vi "bt.vi"(2 "system_stage":string, 8 "LabVIEW Web Service Request":refnum<class "Web Request.lvclass">) -> (1 "position":string, 4 "reduce_head_movement":bool, 7 "congrats_level":string, 9 "therapy_stage":string, 10 "home":string, 13 "target":string, 14 "EEG_Impedances":string, 17 "EOG_Impedances":string, 18 "VI_running":string, 19 "trial_number":string, 26 "VI_stream":string)   [LabVIEW 2020]
uses:
  <vilib>/wsapi/Web Request.lvclass
  Global 1.vi
panel:
  # "Use the Web Service Request input terminal to call the VIs on the Web Services palette. Do not remove it from the connector pane unless you don't need access to the palette."
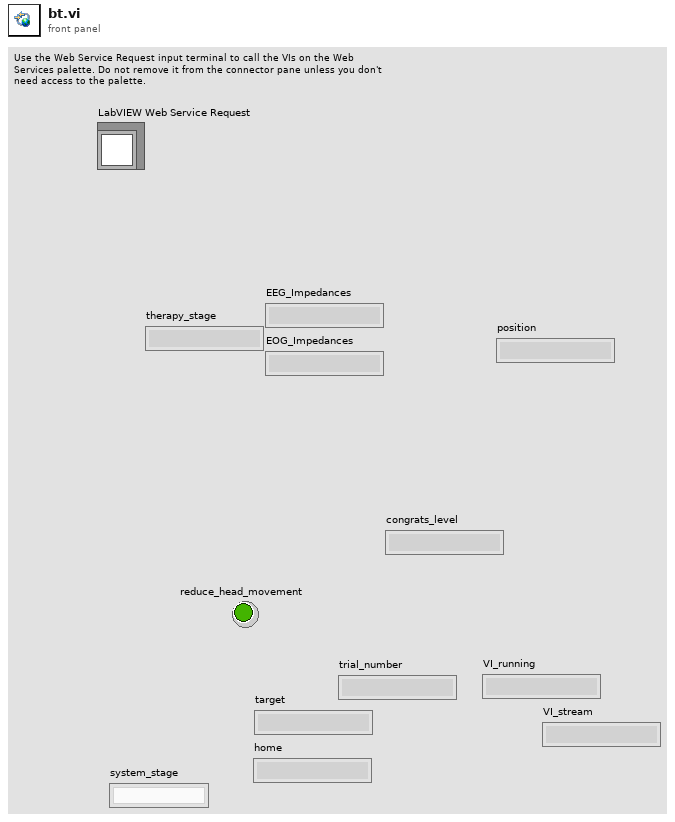
[diagram p1: front panel]
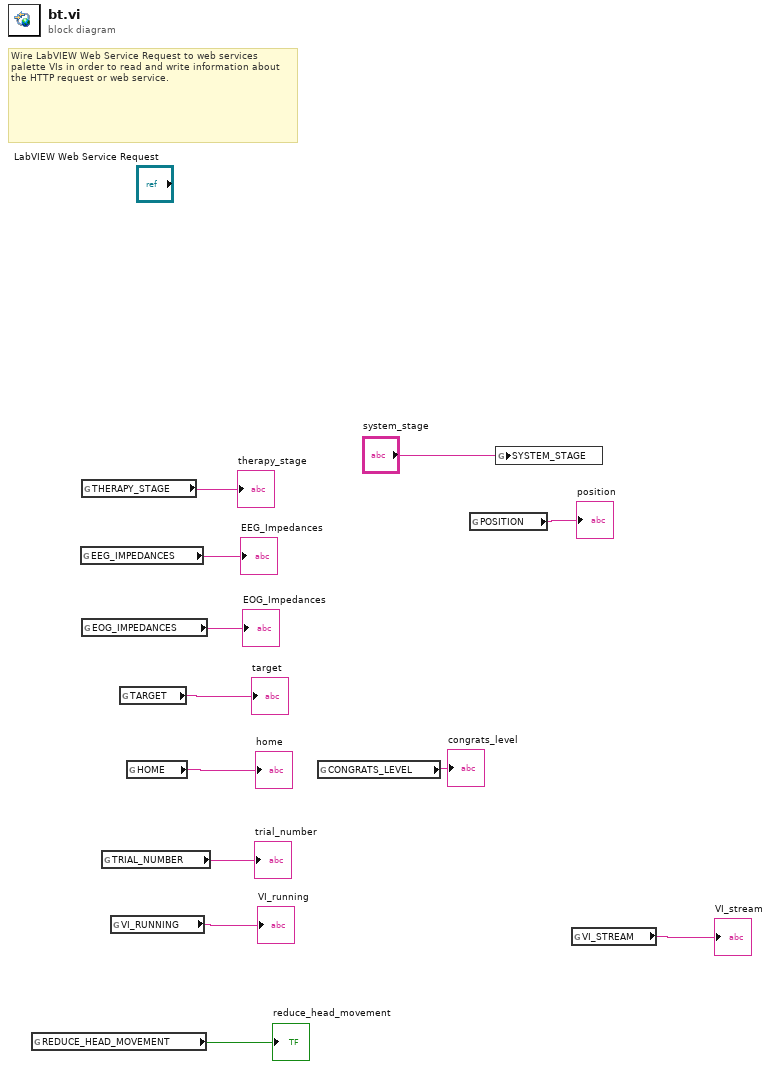
[diagram p0: block diagram]
diagram:
  # "Wire LabVIEW Web Service Request to web services palette VIs in order to read and write information about the HTTP request or web service."
  n1 = global read "Global 1.vi" "REDUCE_HEAD_MOVEMENT"() -> (→"reduce_head_movement":bool)
  n2 = global read "Global 1.vi" "EEG_IMPEDANCES"() -> (→"EEG_Impedances":string)
  n3 = global read "Global 1.vi" "THERAPY_STAGE"() -> (→"therapy_stage":string)
  n4 = global read "Global 1.vi" "EOG_IMPEDANCES"() -> (→"EOG_Impedances":string)
  n5 = global read "Global 1.vi" "TRIAL_NUMBER"() -> (→"trial_number":string)
  n6 = global read "Global 1.vi" "VI_RUNNING"() -> (→"VI_running":string)
  n7 = global read "Global 1.vi" "TARGET"() -> (→"target":string)
  n8 = global read "Global 1.vi" "HOME"() -> (→"home":string)
  n9 = global read "Global 1.vi" "CONGRATS_LEVEL"() -> (→"congrats_level":string)
  n10 = global read "Global 1.vi" "POSITION"() -> (→"position":string)
  n11 = global write "Global 1.vi" "SYSTEM_STAGE"("system_stage") -> ()
  n12 = global read "Global 1.vi" "VI_STREAM"() -> (→"VI_stream":string)
